vi "GetConfigFile.vi"(8 "error in (no error)":errorcluster) -> (0 "error out":errorcluster, 2 "refnum":T1, 3 "section":string="Fanuc SDK parameters")   [LabVIEW 2022 SP3]
uses:
  <vilib>/Utility/config.llb/NI_LVConfig.lvlib
  <vilib>/Utility/config.llb/Config Data RefNum.ctl
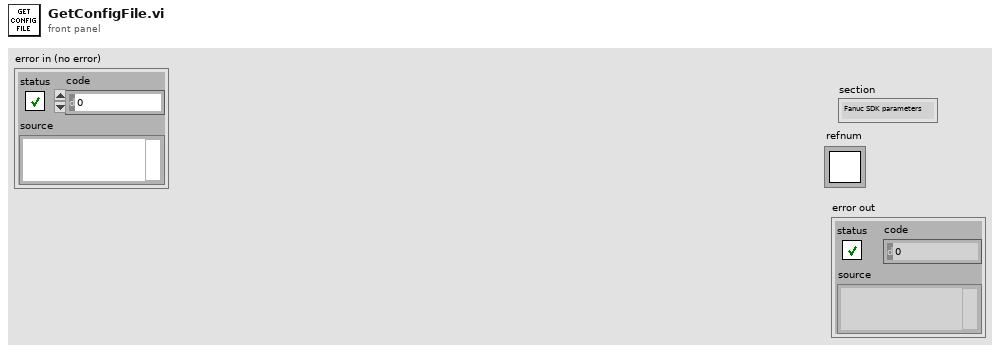
[diagram p1: front panel]
types:
  T1 = typedef "NI_LVConfig.lvlib/Config Data RefNum.ctl" = refnum<k1>
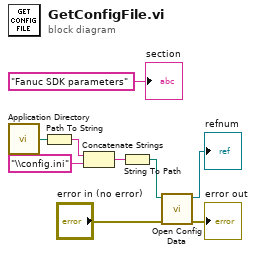
[diagram p0: block diagram]
diagram:
  n1 = call <vilib>:"Application Directory.vi"() -> ("Application Directory"=w9:path)
  n2 = Path To String(path=w9) -> (string=w8:string)
  n3 = Concatenate Strings(w8, "\\config.ini" ("string")) -> (w7:string)
  n4 = String To Path(string=w7) -> (path=w5:path)
  n5 = call <vilib>:"Open Config Data.vi"("error in (no error)"="error in (no error)", "configuration file path"=w5) -> ("error out"=→"error out":errorcluster, "refnum"=→"refnum":T1)  [unwired: 7 in, 1 out]
  "section" <- "Fanuc SDK parameters" ("section")
